vi "volume.get.vi"(8 "error in (no error)":errorcluster, 10 "volume ID":i32, 11 "manager_daemon in":refnum<class "manager_daemon.lvclass">) -> (0 "error out":errorcluster, 2 "volume":T1, 3 "manager_daemon out":refnum<class "manager_daemon.lvclass">)   [LabVIEW 2024, in "manager_daemon.lvclass"]
uses:
  manager_daemon.lvclass
  manager_daemon.lvclass/manager_daemon.ctl
  type_defs/cmd--enum.ctl
  type_defs/msg--cluster.ctl
  CV_Shared_Library/volume.type--enum.ctl
  CV_Shared_Library/CV_Shared_Library.lvlib
  type_defs/VolumeData--cluster.ctl
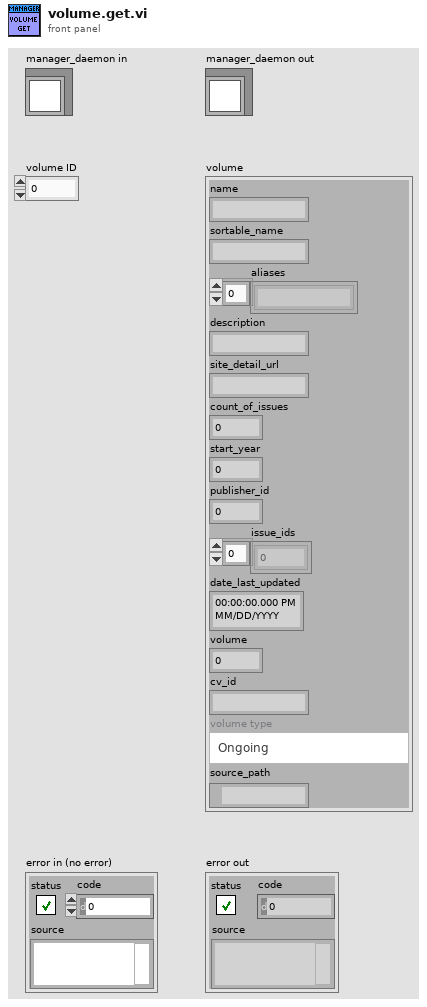
[diagram p1: front panel]
types:
  T1 = typedef "manager_daemon.lvclass/VolumeData--cluster.ctl" = cluster{"name":string, "sortable_name":string, "aliases":string[], "description":string, "site_detail_url":string, "count_of_issues":i32, "start_year":i32, "publisher_id":i32, "issue_ids":i32[], "date_last_updated":timestamp, "volume":i32, "cv_id":string, "volume type":T2, "source_path":path}
  T2 = typedef "CV_Shared_Library.lvlib/volume.type--enum.ctl" = enum16{"Ongoing", "Limited Series", "Annual", "One Shot", "Reprint/Document", "Star Comics", "Epic Comics"}
  T3 = typedef "manager_daemon.lvclass/cmd--enum.ctl" = enum16{"init", "run", "load binaries", "build binaries", "save binaries", "create folder map", "display info", "apply filter", "add volume", "add issues", "add issue", "get volume", "delete volume", "delete issues", "exit"}
  T4 = typedef "manager_daemon.lvclass/msg--cluster.ctl" = cluster{"cmd":T3, "data":variant}
  T5 = cluster{"volume ID":i32, "notifier out":refnum<notifier>}
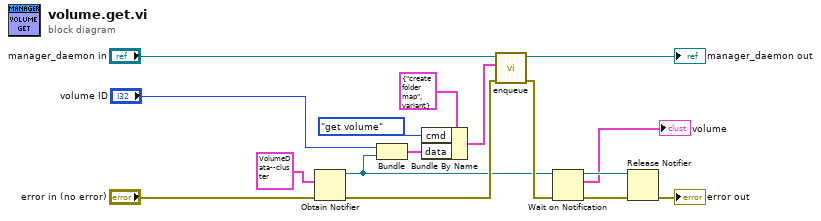
[diagram p0: block diagram]
diagram:
  n1 = Obtain Notifier(notification data type=T1 {"name"="", "sortable_name"="", "aliases"=[], "description"="", "site_detail_url"="", "count_of_issues"=0, "start_year"=0, "publisher_id"=0, "issue_ids"=[], "date_last_updated"=timestamp(0 s since 1904-01-01), "volume"=0, "cv_id"="", "volume type"=enum."Ongoing", "source_path"=path ""} ("value"), error in (no error)="error in (no error)") -> (notifier out=w3:refnum<notifier>, error out=w6:errorcluster)  [unwired: 2 in, 1 out]
  n2 = Bundle("volume ID"="volume ID", "notifier out"=w3) -> (w4:T5)  [unwired: 1 in]
  n3 = Bundle By Name(cluster=T4 {"cmd"=enum."create folder map", "data"=variant} ("msg"), "cmd"=cmd--enum."get volume", "data"=w4) -> (w14:T4)
  n4 = call "enqueue.vi"("error in (no error)"=w6, "msg"=w14, "manager_daemon in"="manager_daemon in") -> ("error out"=w13:errorcluster, "manager_daemon out"=→"manager_daemon out":refnum<class "manager_daemon.lvclass">)  [unwired: 7 in]
  n5 = Wait on Notification(notifier=w3, error in (no error)=w13) -> (notifier out=w11:refnum<notifier>, notification=→"volume":T1, error out=w10:errorcluster)  [unwired: 2 in, 1 out]
  n6 = Release Notifier(notifier=w11, error in (no error)=w10) -> (error out=→"error out":errorcluster)  [unwired: 1 in, 2 out]
